vi "main.vi"() -> ()   [LabVIEW 2023] (continued)
     4245  0CF104A7   00000004    8        F0\t60\t22\tFC\tFF\tFF\tFF\t62\r\n      4244  0CF103A7   00000004    8        17\t1F\t08\t60\tB1\t1F\t08\t62\r\n      4244  0CF102A7   00000004    8        30\t75\tE0\t2E\t80\tFF\tFF\tFD\r\n      4243  0C3C4D4A   00000004    8        BE\tFF\tFF\t7F\t18\tFF\tFF\t62\r\n      4243  0CF101A7   00000004    8        68\t00\t97\tCC\t00\t19\t39\tEE\r\n      4242  18F120F0   00000004    8        2B\t75\t60\tB1\tB0\t01\tFF\tFF\r\n      4241  18F11FF0   00000004    8        FF\t3F\t90\t68\t88\t1B\t10\t2C\r\n      4232  1FFFFFFF   00000004    8        00\t20\tFF\tFF\tFF\tFF\tFF\tFF\r\n      4223  0CF102A7   00000004    8        30\t75\tE0\t2E\t80\tFF\tFF\tFD\r\n      4223  0CF101A7   00000004    8        68\t00\t97\tCC\t00\t19\t39\tED\r\n      4246  18F121F0   00000004    8        09\t34\t00\t00\tFF\tFF\tB0\t01\r\n      4245  18F106A7   00000004    8        00\tF7\tFF\tFF\tFF\tFF\tFF\tC5\r\n      4245  0CF104A7   00000004    8        F0\t60\t22\tFC\tFF\tFF\tFF\t62\r\n      4244  0CF103A7   00000004    8        17\t1F\t08\t60\tB1\t1F\t08\t62\r\n      4244  0CF102A7   00000004    8        30\t75\tE0\t2E\t80\tFF\tFF\tFD\r\n      4243  0C3C4D4A   00000004    8        BE\tFF\tFF\t7F\t18\tFF\tFF\t62\r\n      4243  0CF101A7   00000004    8        68\t00\t97\tCC\t00\t19\t39\tEE\r\n      4242  18F120F0   00000004    8        2B\t75\t60\tB1\tB0\t01\tFF\tFF\r\n      4241  18F11FF0   00000004    8        FF\t3F\t90\t68\t88\t1B\t10\t2C\r\n      4232  1FFFFFFF   00000004    8        00\t20\tFF\tFF\tFF\tFF\tFF\tFF\r\n      4223  0CF102A7   00000004    8        30\t75\tE0\t2E\t80\tFF\tFF\tFD\r\n      4247  1FFFFFFF   00000004    8        00\t00\tFF\tFF\tFF\tFF\tFF\tFF\r\n      4246  18F121F0   00000004    8        09\t34\t00\t00\tFF\tFF\tB0\t01\r\n      4245  18F106A7   00000004    8        00\tF7\tFF\tFF\tFF\tFF\tFF\tC5\r\n      4245  0CF104A7   00000004    8        F0\t60\t22\tFC\tFF\tFF\tFF\t62\r\n      4244  0CF103A7   00000004    8        17\t1F\t08\t60\tB1\t1F\t08\t62\r\n      4244  0CF102A7   00000004    8        30\t75\tE0\t2E\t80\tFF\tFF\tFD\r\n      4243  0C3C4D4A   00000004    8        BE\tFF\tFF\t7F\t18\tFF\tFF\t62\r\n      4243  0CF101A7   00000004    8        68\t00\t97\tCC\t00\t19\t39\tEE\r\n      4242  18F120F0   00000004    8        2B\t75\t60\tB1\tB0\t01\tFF\tFF\r\n      4241  18F11FF0   00000004    8        FF\t3F\t90\t68\t88\t1B\t10\t2C\r\n      4232  1FFFFFFF   00000004    8        00\t20\tFF\tFF\tFF\tFF\tFF\tFF\r\n      4252  1FFFFFFF   00000004    8        00\t20\tFF\tFF\tFF\tFF\tFF\tFF\r\n      4247  1FFFFFFF   00000004    8        00\t00\tFF\tFF\tFF\tFF\tFF\tFF\r\n      4246  18F121F0   00000004    8        09\t34\t00\t00\tFF\tFF\tB0\t01\r\n      4245  18F106A7   00000004    8        00\tF7\tFF\tFF\tFF\tFF\tFF\tC5\r\n      4245  0CF104A7   00000004    8        F0\t60\t22\tFC\tFF\tFF\tFF\t62\r\n      4244  0CF103A7   00000004    8        17\t1F\t08\t60\tB1\t1F\t08\t62\r\n      4244  0CF102A7   00000004    8        30\t75\tE0\t2E\t80\tFF\tFF\tFD\r\n      4243  0C3C4D4A   00000004    8        BE\tFF\tFF\t7F\t18\tFF\tFF\t62\r\n      4243  0CF101A7   00000004    8        68\t00\t97\tCC\t00\t19\t39\tEE\r\n      4242  18F120F0   00000004    8        2B\t75\t60\tB1\tB0\t01\tFF\tFF\r\n      4241  18F11FF0   00000004    8        FF\t3F\t90\t68\t88\t1B\t10\t2C\r\n      4262  1FFFFFFF   00000004    8        00\t20\tFF\tFF\tFF\tFF\tFF\tFF\r\n      4252  1FFFFFFF   00000004    8        00\t20\tFF\tFF\tFF\tFF\tFF\tFF\r\n      4247  1FFFFFFF   00000004    8        00\t00\tFF\tFF\tFF\tFF\tFF\tFF\r\n      4246  18F121F0   00000004    8        09\t34\t00\t00\tFF\tFF\tB0\t01\r\n      4245  18F106A7   00000004    8        00\tF7\tFF\tFF\tFF\tFF\tFF\tC5\r\n      4245  0CF104A7   00000004    8        F0\t60\t22\tFC\tFF\tFF\tFF\t62\r\n      4244  0CF103A7   00000004    8        17\t1F\t08\t60\tB1\t1F\t08\t62\r\n      4244  0CF102A7   00000004    8        30\t75\tE0\t2E\t80\tFF\tFF\tFD\r\n      4243  0C3C4D4A   00000004    8        BE\tFF\tFF\t7F\t18\tFF\tFF\t62\r\n      4243  0CF101A7   00000004    8        68\t00\t97\tCC\t00\t19\t39\tEE\r\n      4242  18F120F0   00000004    8        2B\t75\t60\tB1\tB0\t01\tFF\tFF\r\n      4263  0CF101A7   00000004    8        68\t00\t97\tCC\t00\t19\t39\tEF\r\n      4262  1FFFFFFF   00000004    8        00\t20\tFF\tFF\tFF\tFF\tFF\tFF\r\n      4252  1FFFFFFF   00000004    8        00\t20\tFF\tFF\tFF\tFF\tFF\tFF\r\n      4247  1FFFFFFF   00000004    8        00\t00\tFF\tFF\tFF\tFF\tFF\tFF\r\n      4246  18F121F0   00000004    8        09\t34\t00\t00\tFF\tFF\tB0\t01\r\n      4245  18F106A7   00000004    8        00\tF7\tFF\tFF\tFF\tFF\tFF\tC5\r\n      4245  0CF104A7   00000004    8        F0\t60\t22\tFC\tFF\tFF\tFF\t62\r\n      4244  0CF103A7   00000004    8        17\t1F\t08\t60\tB1\t1F\t08\t62\r\n      4244  0CF102A7   00000004    8        30\t75\tE0\t2E\t80\tFF\tFF\tFD\r\n      4243  0C3C4D4A   00000004    8        BE\tFF\tFF\t7F\t18\tFF\tFF\t62\r\n      4243  0CF101A7   00000004    8        68\t00\t97\tCC\t00\t19\t39\tEE\r\n      4263  0CF102A7   00000004    8        30\t75\tE0\t2E\t80\tFF\tFF\tFD\r\n      4263  0CF101A7   00000004    8        68\t00\t97\tCC\t00\t19\t39\tEF\r\n      4262  1FFFFFFF   00000004    8        00\t20\tFF\tFF\tFF\tFF\tFF\tFF\r\n      4252  1FFFFFFF   00000004    8        00\t20\tFF\tFF\tFF\tFF\tFF\tFF\r\n      4247  1FFFFFFF   00000004    8        00\t00\tFF\tFF\tFF\tFF\tFF\tFF\r\n      4246  18F121F0   00000004    8        09\t34\t00\t00\tFF\tFF\tB0\t01\r\n      4245  18F106A7   00000004    8        00\tF7\tFF\tFF\tFF\tFF\tFF\tC5\r\n      4245  0CF104A7   00000004    8        F0\t60\t22\tFC\tFF\tFF\tFF\t62\r\n      4244  0CF103A7   00000004    8        17\t1F\t08\t60\tB1\t1F\t08\t62\r\n      4244  0CF102A7   00000004    8        30\t75\tE0\t2E\t80\tFF\tFF\tFD\r\n      4243  0C3C4D4A   00000004    8        BE\tFF\tFF\t7F\t18\tFF\tFF\t62\r\n      4272  1FFFFFFF   00000004    8        00\t00\tFF\tFF\tFF\tFF\tFF\tFF\r\n      4263  0CF102A7   00000004    8        30\t75\tE0\t2E\t80\tFF\tFF\tFD\r\n      4263  0CF101A7   00000004    8        68\t00\t97\tCC\t00\t19\t39\tEF\r\n      4262  1FFFFFFF   00000004    8        00\t20\tFF\tFF\tFF\tFF\tFF\tFF\r\n      4252  1FFFFFFF   00000004    8        00\t20\tFF\tFF\tFF\tFF\tFF\tFF\r\n      4247  1FFFFFFF   00000004    8        00\t00\tFF\tFF\tFF\tFF\tFF\tFF\r\n      4246  18F121F0   00000004    8        09\t34\t00\t00\tFF\tFF\tB0\t01\r\n      4245  18F106A7   00000004    8        00\tF7\tFF\tFF\tFF\tFF\tFF\tC5\r\n      4245  0CF104A7   00000004    8        F0\t60\t22\tFC\tFF\tFF\tFF\t62\r\n      4244  0CF103A7   00000004    8        17\t1F\t08\t60\tB1\t1F\t08\t62\r\n      4244  0CF102A7   00000004    8        30\t75\tE0\t2E\t80\tFF\tFF\tFD\r\n      4282  1FFFFFFF   00000004    8        00\t00\tFF\tFF\tFF\tFF\tFF\tFF\r\n      4272  1FFFFFFF   00000004    8        00\t00\tFF\tFF\tFF\tFF\tFF\tFF\r\n      4263  0CF102A7   00000004    8        30\t75\tE0\t2E\t80\tFF\tFF\tFD\r\n      4263  0CF101A7   00000004    8        68\t00\t97\tCC\t00\t19\t39\tEF\r\n      4262  1FFFFFFF   00000004    8        00\t20\tFF\tFF\tFF\tFF\tFF\tFF\r\n      4252  1FFFFFFF   00000004    8        00\t20\tFF\tFF\tFF\tFF\tFF\tFF\r\n      4247  1FFFFFFF   00000004    8        00\t00\tFF\tFF\tFF\tFF\tFF\tFF\r\n      4246  18F121F0   00000004    8        09\t34\t00\t00\tFF\tFF\tB0\t01\r\n      4245  18F106A7   00000004    8        00\tF7\tFF\tFF\tFF\tFF\tFF\tC5\r\n      4245  0CF104A7   00000004    8        F0\t60\t22\tFC\tFF\tFF\tFF\t62\r\n      4244  0CF103A7   00000004    8        17\t1F\t08\t60\tB1\t1F\t08\t62\r\n      4283  0CF101A7   00000004    8        68\t00\t97\tCC\t00\t19\t39\tF0\r\n      4282  1FFFFFFF   00000004    8        00\t00\tFF\tFF\tFF\tFF\tFF\tFF\r\n      4272  1FFFFFFF   00000004    8        00\t00\tFF\tFF\tFF\tFF\tFF\tFF\r\n      4263  0CF102A7   00000004    8        30\t75\tE0\t2E\t80\tFF\tFF\tFD\r\n      4263  0CF101A7   00000004    8        68\t00\t97\tCC\t00\t19\t39\tEF\r\n      4262  1FFFFFFF   00000004    8        00\t20\tFF\tFF\tFF\tFF\tFF\tFF\r\n      4252  1FFFFFFF   00000004    8        00\t20\tFF\tFF\tFF\tFF\tFF\tFF\r\n      4247  1FFFFFFF   00000004    8        00\t00\tFF\tFF\tFF\tFF\tFF\tFF\r\n      4246  18F121F0   00000004    8        09\t34\t00\t00\tFF\tFF\tB0\t01\r\n      4245  18F106A7   00000004    8        00\tF7\tFF\tFF\tFF\tFF\tFF\tC5\r\n      4245  0CF104A7   00000004    8        F0\t60\t22\tFC\tFF\tFF\tFF\t62\r\n      4283  0CF102A7   00000004    8        30\t75\tE0\t2E\t80\tFF\tFF\tFD\r\n      4283  0CF101A7   00000004    8        68\t00\t97\tCC\t00\t19\t39\tF0\r\n      4282  1FFFFFFF   00000004    8        00\t00\tFF\tFF\tFF\tFF\tFF\tFF\r\n      4272  1FFFFFFF   00000004    8        00\t00\tFF\tFF\tFF\tFF\tFF\tFF\r\n      4263  0CF102A7   00000004    8        30\t75\tE0\t2E\t80\tFF\tFF\tFD\r\n      4263  0CF101A7   00000004    8        68\t00\t97\tCC\t00\t19\t39\tEF\r\n      4262  1FFFFFFF   00000004    8        00\t20\tFF\tFF\tFF\tFF\tFF\tFF\r\n      4252  1FFFFFFF   00000004    8        00\t20\tFF\tFF\tFF\tFF\tFF\tFF\r\n      4247  1FFFFFFF   00000004    8        00\t00\tFF\tFF\tFF\tFF\tFF\tFF\r\n      4246  18F121F0   00000004    8        09\t34\t00\t00\tFF\tFF\tB0\t01\r\n      4245  18F106A7   00000004    8        00\tF7\tFF\tFF\tFF\tFF\tFF\tC5\r\n      4292  1FFFFFFF   00000004    8        00\t20\tFF\tFF\tFF\tFF\tFF\tFF\r\n      4283  0CF102A7   00000004    8        30\t75\tE0\t2E\t80\tFF\tFF\tFD\r\n      4283  0CF101A7   00000004    8        68\t00\t97\tCC\t00\t19\t39\tF0\r\n      4282  1FFFFFFF   00000004    8        00\t00\tFF\tFF\tFF\tFF\tFF\tFF\r\n      4272  1FFFFFFF   00000004    8        00\t00\tFF\tFF\tFF\tFF\tFF\tFF\r\n      4263  0CF102A7   00000004    8        30\t75\tE0\t2E\t80\tFF\tFF\tFD\r\n      4263  0CF101A7   00000004    8        68\t00\t97\tCC\t00\t19\t39\tEF\r\n      4262  1FFFFFFF   00000004    8        00\t20\tFF\tFF\tFF\tFF\tFF\tFF\r\n      4252  1FFFFFFF   00000004    8        00\t20\tFF\tFF\tFF\tFF\tFF\tFF\r\n      4247  1FFFFFFF   00000004    8        00\t00\tFF\tFF\tFF\tFF\tFF\tFF\r\n      4246  18F121F0   00000004    8        09\t34\t00\t00\tFF\tFF\tB0\t01\r\n      4293  18F106A7   00000004    8        00\tF7\tFF\tFF\tFF\tFF\tFF\tC6\r\n      4292  1FFFFFFF   00000004    8        00\t20\tFF\tFF\tFF\tFF\tFF\tFF\r\n      4283  0CF102A7   00000004    8        30\t75\tE0\t2E\t80\tFF\tFF\tFD\r\n      4283  0CF101A7   00000004    8        68\t00\t97\tCC\t00\t19\t39\tF0\r\n      4282  1FFFFFFF   00000004    8        00\t00\tFF\tFF\tFF\tFF\tFF\tFF\r\n      4272  1FFFFFFF   00000004    8        00\t00\tFF\tFF\tFF\tFF\tFF\tFF\r\n      4263  0CF102A7   00000004    8        30\t75\tE0\t2E\t80\tFF\tFF\tFD\r\n      4263  0CF101A7   00000004    8        68\t00\t97\tCC\t00\t19\t39\tEF\r\n      4262  1FFFFFFF   00000004    8        00\t20\tFF\tFF\tFF\tFF\tFF\tFF\r\n      4252  1FFFFFFF   00000004    8        00\t20\tFF\tFF\tFF\tFF\tFF\tFF\r\n      4247  1FFFFFFF   00000004    8        00\t00\tFF\tFF\tFF\tFF\tFF\tFF\r\n      4302  1FFFFFFF   00000004    8        00\t00\tFF\tFF\tFF\tFF\tFF\tFF\r\n      4293  18F106A7   00000004    8        00\tF7\tFF\tFF\tFF\tFF\tFF\tC6\r\n      4292  1FFFFFFF   00000004    8        00\t20\tFF\tFF\tFF\tFF\tFF\tFF\r\n      4283  0CF102A7   00000004    8        30\t75\tE0\t2E\t80\tFF\tFF\tFD\r\n      4283  0CF101A7   00000004    8        68\t00\t97\tCC\t00\t19\t39\tF0\r\n      4282  1FFFFFFF   00000004    8        00\t00\tFF\tFF\tFF\tFF\tFF\tFF\r\n      4272  1FFFFFFF   00000004    8        00\t00\tFF\tFF\tFF\tFF\tFF\tFF\r\n      4263  0CF102A7   00000004    8        30\t75\tE0\t2E\t80\tFF\tFF\tFD\r\n      4263  0CF101A7   00000004    8        68\t00\t97\tCC\t00\t19\t39\tEF\r\n      4262  1FFFFFFF   00000004    8        00\t20\tFF\tFF\tFF\tFF\tFF\tFF\r\n      4252  1FFFFFFF   00000004    8        00\t20\tFF\tFF\tFF\tFF\tFF\tFF\r\n      4303  0CF101A7   00000004    8        68\t00\t97\tCC\t00\t19\t39\tF1\r\n      4302  1FFFFFFF   00000004    8        00\t00\tFF\tFF\tFF\tFF\tFF\tFF\r\n      4293  18F106A7   00000004    8        00\tF7\tFF\tFF\tFF\tFF\tFF\tC6\r\n      4292  1FFFFFFF   00000004    8        00\t20\tFF\tFF\tFF\tFF\tFF\tFF\r\n      4283  0CF102A7   00000004    8        30\t75\tE0\t2E\t80\tFF\tFF\tFD\r\n      4283  0CF101A7   00000004    8        68\t00\t97\tCC\t00\t19\t39\tF0\r\n      4282  1FFFFFFF   00000004    8        00\t00\tFF\tFF\tFF\tFF\tFF\tFF\r\n      4272  1FFFFFFF   00000004    8        00\t00\tFF\tFF\tFF\tFF\tFF\tFF\r\n      4263  0CF102A7   00000004    8        30\t75\tE0\t2E\t80\tFF\tFF\tFD\r\n      4263  0CF101A7   00000004    8        68\t00\t97\tCC\t00\t19\t39\tEF\r\n      4262  1FFFFFFF   00000004    8        00\t20\tFF\tFF\tFF\tFF\tFF\tFF\r\n      4303  0CF102A7   00000004    8        30\t75\tE0\t2E\t80\tFF\tFF\tFD\r\n      4303  0CF101A7   00000004    8        68\t00\t97\tCC\t00\t19\t39\tF1\r\n      4302  1FFFFFFF   00000004    8        00\t00\tFF\tFF\tFF\tFF\tFF\tFF\r\n      4293  18F106A7   00000004    8        00\tF7\tFF\tFF\tFF\tFF\tFF\tC6\r\n      4292  1FFFFFFF   00000004    8        00\t20\tFF\tFF\tFF\tFF\tFF\tFF\r\n      4283  0CF102A7   00000004    8        30\t75\tE0\t2E\t80\tFF\tFF\tFD\r\n      4283  0CF101A7   00000004    8        68\t00\t97\tCC\t00\t19\t39\tF0\r\n      4282  1FFFFFFF   00000004    8        00\t00\tFF\tFF\tFF\tFF\tFF\tFF\r\n      4272  1FFFFFFF   00000004    8        00\t00\tFF\tFF\tFF\tFF\tFF\tFF\r\n      4263  0CF102A7   00000004    8        30\t75\tE0\t2E\t80\tFF\tFF\tFD\r\n      4263  0CF101A7   00000004    8        68\t00\t97\tCC\t00\t19\t39\tEF\r\n      4312  1FFFFFFF   00000004    8        00\t20\tFF\tFF\tFF\tFF\tFF\tFF\r\n      4303  0CF102A7   00000004    8        30\t75\tE0\t2E\t80\tFF\tFF\tFD\r\n      4303  0CF101A7   00000004    8        68\t00\t97\tCC\t00\t19\t39\tF1\r\n      4302  1FFFFFFF   00000004    8        00\t00\tFF\tFF\tFF\tFF\tFF\tFF\r\n      4293  18F106A7   00000004    8        00\tF7\tFF\tFF\tFF\tFF\tFF\tC6\r\n      4292  1FFFFFFF   00000004    8        00\t20\tFF\tFF\tFF\tFF\tFF\tFF\r\n      4283  0CF102A7   00000004    8        30\t75\tE0\t2E\t80\tFF\tFF\tFD\r\n      4283  0CF101A7   00000004    8        68\t00\t97\tCC\t00\t19\t39\tF0\r\n      4282  1FFFFFFF   00000004    8        00\t00\tFF\tFF\tFF\tFF\tFF\tFF\r\n      4272  1FFFFFFF   00000004    8        00\t00\tFF\tFF\tFF\tFF\tFF\tFF\r\n      4263  0CF102A7   00000004    8        30\t75\tE0\t2E\t80\tFF\tFF\tFD\r\n      4322  1FFFFFFF   00000004    8        00\t00\tFF\tFF\tFF\tFF\tFF\tFF\r\n      4312  1FFFFFFF   00000004    8        00\t20\tFF\tFF\tFF\tFF\tFF\tFF\r\n      4303  0CF102A7   00000004    8        30\t75\tE0\t2E\t80\tFF\tFF\tFD\r\n      4303  0CF101A7   00000004    8        68\t00\t97\tCC\t00\t19\t39\tF1\r\n      4302  1FFFFFFF   00000004    8        00\t00\tFF\tFF\tFF\tFF\tFF\tFF\r\n      4293  18F106A7   00000004    8        00\tF7\tFF\tFF\tFF\tFF\tFF\tC6\r\n      4292  1FFFFFFF   00000004    8        00\t20\tFF\tFF\tFF\tFF\tFF\tFF\r\n      4283  0CF102A7   00000004    8        30\t75\tE0\t2E\t80\tFF\tFF\tFD\r\n      4283  0CF101A7   00000004    8        68\t00\t97\tCC\t00\t19\t39\tF0\r\n      4282  1FFFFFFF   00000004    8        00\t00\tFF\tFF\tFF\tFF\tFF\tFF\r\n      4272  1FFFFFFF   00000004    8        00\t00\tFF\tFF\tFF\tFF\tFF\tFF\r\n      4322  0CF101A7   00000004    8        68\t00\t97\tCC\t00\t19\t39\tF2\r\n      4322  1FFFFFFF   00000004    8        00\t00\tFF\tFF\tFF\tFF\tFF\tFF\r\n      4312  1FFFFFFF   00000004    8        00\t20\tFF\tFF\tFF\tFF\tFF\tFF\r\n      4303  0CF102A7   00000004    8        30\t75\tE0\t2E\t80\tFF\tFF\tFD\r\n      4303  0CF101A7   00000004    8        68\t00\t97\tCC\t00\t19\t39\tF1\r\n      4302  1FFFFFFF   00000004    8        00\t00\tFF\tFF\tFF\tFF\tFF\tFF\r\n      4293  18F106A7   00000004    8        00\tF7\tFF\tFF\tFF\tFF\tFF\tC6\r\n      4292  1FFFFFFF   00000004    8        00\t20\tFF\tFF\tFF\tFF\tFF\tFF\r\n      4283  0CF102A7   00000004    8        30\t75\tE0\t2E\t80\tFF\tFF\tFD\r\n      4283  0CF101A7   00000004    8        68\t00\t97\tCC\t00\t19\t39\tF0\r\n      4282  1FFFFFFF   00000004    8        00\t00\tFF\tFF\tFF\tFF\tFF\tFF\r\n      4323  0CF102A7   00000004    8        30\t75\tE0\t2E\t80\tFF\tFF\tFD\r\n      4322  0CF101A7   00000004    8        68\t00\t97\tCC\t00\t19\t39\tF2\r\n      4322  1FFFFFFF   00000004    8        00\t00\tFF\tFF\tFF\tFF\tFF\tFF\r\n      4312  1FFFFFFF   00000004    8        00\t20\tFF\tFF\tFF\tFF\tFF\tFF\r\n      4303  0CF102A7   00000004    8        30\t75\tE0\t2E\t80\tFF\tFF\tFD\r\n      4303  0CF101A7   00000004    8        68\t00\t97\tCC\t00\t19\t39\tF1\r\n      4302  1FFFFFFF   00000004    8        00\t00\tFF\tFF\tFF\tFF\tFF\tFF\r\n      4293  18F106A7   00000004    8        00\tF7\tFF\tFF\tFF\tFF\tFF\tC6\r\n      4292  1FFFFFFF   00000004    8        00\t20\tFF\tFF\tFF\tFF\tFF\tFF\r\n      4283  0CF102A7   00000004    8        30\t75\tE0\t2E\t80\tFF\tFF\tFD\r\n      4283  0CF101A7   00000004    8        68\t00\t97\tCC\t00\t19\t39\tF0\r\n      4332  1FFFFFFF   00000004    8        00\t20\tFF\tFF\tFF\tFF\tFF\tFF\r\n      4323  0CF102A7   00000004    8        30\t75\tE0\t2E\t80\tFF\tFF\tFD\r\n      4322  0CF101A7   00000004    8        68\t00\t97\tCC\t00\t19\t39\tF2\r\n      4322  1FFFFFFF   00000004    8        00\t00\tFF\tFF\tFF\tFF\tFF\tFF\r\n      4312  1FFFFFFF   00000004    8        00\t20\tFF\tFF\tFF\tFF\tFF\tFF\r\n      4303  0CF102A7   00000004    8        30\t75\tE0\t2E\t80\tFF\tFF\tFD\r\n      4303  0CF101A7   00000004    8        68\t00\t97\tCC\t00\t19\t39\tF1\r\n      4302  1FFFFFFF   00000004    8        00\t00\tFF\tFF\tFF\tFF\tFF\tFF\r\n      4293  18F106A7   00000004    8        00\tF7\tFF\tFF\tFF\tFF\tFF\tC6\r\n      4292  1FFFFFFF   00000004    8        00\t20\tFF\tFF\tFF\tFF\tFF\tFF\r\n      4283  0CF102A7   00000004    8        30\t75\tE0\t2E\t80\tFF\tFF\tFD\r\n      4341  18F11FF0   00000004    8        FF\t3F\t90\t68\t88\t1B\t10\t3C\r\n      4332  1FFFFFFF   00000004    8        00\t20\tFF\tFF\tFF\tFF\tFF\tFF\r\n      4323  0CF102A7   00000004    8        30\t75\tE0\t2E\t80\tFF\tFF\tFD\r\n      4322  0CF101A7   00000004    8        68\t00\t97\tCC\t00\t19\t39\tF2\r\n      4322  1FFFFFFF   00000004    8        00\t00\tFF\tFF\tFF\tFF\tFF\tFF\r\n      4312  1FFFFFFF   00000004    8        00\t20\tFF\tFF\tFF\tFF\tFF\tFF\r\n      4303  0CF102A7   00000004    8        30\t75\tE0\t2E\t80\tFF\tFF\tFD\r\n      4303  0CF101A7   00000004    8        68\t00\t97\tCC\t00\t19\t39\tF1\r\n      4302  1FFFFFFF   00000004    8        00\t00\tFF\tFF\tFF\tFF\tFF\tFF\r\n      4293  18F106A7   00000004    8        00\tF7\tFF\tFF\tFF\tFF\tFF\tC6\r\n      4292  1FFFFFFF   00000004    8        00\t20\tFF\tFF\tFF\tFF\tFF\tFF\r\n      4342  18F120F0   00000004    8        2B\t75\t60\tB1\tB0\t01\tFF\tFF\r\n      4341  18F11FF0   00000004    8        FF\t3F\t90\t68\t88\t1B\t10\t3C\r\n      4332  1FFFFFFF   00000004    8        00\t20\tFF\tFF\tFF\tFF\tFF\tFF\r\n      4323  0CF102A7   00000004    8        30\t75\tE0\t2E\t80\tFF\tFF\tFD\r\n      4322  0CF101A7   00000004    8        68\t00\t97\tCC\t00\t19\t39\tF2\r\n      4322  1FFFFFFF   00000004    8        00\t00\tFF\tFF\tFF\tFF\tFF\tFF\r\n      4312  1FFFFFFF   00000004    8        00\t20\tFF\tFF\tFF\tFF\tFF\tFF\r\n      4303  0CF102A7   00000004    8        30\t75\tE0\t2E\t80\tFF\tFF\tFD\r\n      4303  0CF101A7   00000004    8        68\t00\t97\tCC\t00\t19\t39\tF1\r\n      4302  1FFFFFFF   00000004    8        00\t00\tFF\tFF\tFF\tFF\tFF\tFF\r\n      4293  18F106A7   00000004    8        00\tF7\tFF\tFF\tFF\tFF\tFF\tC6\r\n      4343  0CF101A7   00000004    8        68\t00\t97\tCC\t00\t19\t39\tF3\r\n      4342  18F120F0   00000004    8        2B\t75\t60\tB1\tB0\t01\tFF\tFF\r\n      4341  18F11FF0   00000004    8        FF\t3F\t90\t68\t88\t1B\t10\t3C\r\n      4332  1FFFFFFF   00000004    8        00\t20\tFF\tFF\tFF\tFF\tFF\tFF\r\n      4323  0CF102A7   00000004    8        30\t75\tE0\t2E\t80\tFF\tFF\tFD\r\n      4322  0CF101A7   00000004    8        68\t00\t97\tCC\t00\t19\t39\tF2\r\n      4322  1FFFFFFF   00000004    8        00\t00\tFF\tFF\tFF\tFF\tFF\tFF\r\n      4312  1FFFFFFF   00000004    8        00\t20\tFF\tFF\tFF\tFF\tFF\tFF\r\n      4303  0CF102A7   00000004    8        30\t75\tE0\t2E\t80\tFF\tFF\tFD\r\n      4303  0CF101A7   00000004    8        68\t00\t97\tCC\t00\t19\t39\tF1\r\n      4302  1FFFFFFF   00000004    8        00\t00\tFF\tFF\tFF\tFF\tFF\tFF\r\n      4343  0C3C4D4A   00000004    8        BE\tFF\tFF\t7F\t18\tFF\tFF\t63\r\n      4343  0CF101A7   00000004    8        68\t00\t97\tCC\t00\t19\t39\tF3\r\n      4342  18F120F0   00000004    8        2B\t75\t60\tB1\tB0\t01\tFF\tFF\r\n      4341  18F11FF0   00000004    8        FF\t3F\t90\t68\t88\t1B\t10\t3C\r\n      4332  1FFFFFFF   00000004    8        00\t20\tFF\tFF\tFF\tFF\tFF\tFF\r\n      4323  0CF102A7   00000004    8        30\t75\tE0\t2E\t80\tFF\tFF\tFD\r\n      4322  0CF101A7   00000004    8        68\t00\t97\tCC\t00\t19\t39\tF2\r\n      4322  1FFFFFFF   00000004    8        00\t00\tFF\tFF\tFF\tFF\tFF\tFF\r\n      4312  1FFFFFFF   00000004    8        00\t20\tFF\tFF\tFF\tFF\tFF\tFF\r\n      4303  0CF102A7   00000004    8        30\t75\tE0\t2E\t80\tFF\tFF\tFD\r\n      4303  0CF101A7   00000004    8        68\t00\t97\tCC\t00\t19\t39\tF1\r\n      4344  0CF102A7   00000004    8        30\t75\tE0\t2E\t80\tFF\tFF\tFD\r\n      4343  0C3C4D4A   00000004    8        BE\tFF\tFF\t7F\t18\tFF\tFF\t63\r\n      4343  0CF101A7   00000004    8        68\t00\t97\tCC\t00\t19\t39\tF3\r\n      4342  18F120F0   00000004    8        2B\t75\t60\tB1\tB0\t01\tFF\tFF\r\n      4341  18F11FF0   00000004    8        FF\t3F\t90\t68\t88\t1B\t10\t3C\r\n      4332  1FFFFFFF   00000004    8        00\t20\tFF\tFF\tFF\tFF\tFF\tFF\r\n      4323  0CF102A7   00000004    8        30\t75\tE0\t2E\t80\tFF\tFF\tFD\r\n      4322  0CF101A7   00000004    8        68\t00\t97\tCC\t00\t19\t39\tF2\r\n      4322  1FFFFFFF   00000004    8        00\t00\tFF\tFF\tFF\tFF\tFF\tFF\r\n      4312  1FFFFFFF   00000004    8        00\t20\tFF\tFF\tFF\tFF\tFF\tFF\r\n      4303  0CF102A7   00000004    8        30\t75\tE0\t2E\t80\tFF\tFF\tFD\r\n      4344  0CF103A7   00000004    8        17\t1F\t08\t60\tB1\t1F\t08\t63\r\n      4344  0CF102A7   00000004    8        30\t75\tE0\t2E\t80\tFF\tFF\tFD\r\n      4343  0C3C4D4A   00000004    8        BE\tFF\tFF\t7F\t18\tFF\tFF\t63\r\n      4343  0CF101A7   00000004    8        68\t00\t97\tCC\t00\t19\t39\tF3\r\n      4342  18F120F0   00000004    8        2B\t75\t60\tB1\tB0\t01\tFF\tFF\r\n      4341  18F11FF0   00000004    8        FF\t3F\t90\t68\t88\t1B\t10\t3C\r\n      4332  1FFFFFFF   00000004    8        00\t20\tFF\tFF\tFF\tFF\tFF\tFF\r\n      4323  0CF102A7   00000004    8        30\t75\tE0\t2E\t80\tFF\tFF\tFD\r\n      4322  0CF101A7   00000004    8        68\t00\t97\tCC\t00\t19\t39\tF2\r\n      4322  1FFFFFFF   00000004    8        00\t00\tFF\tFF\tFF\tFF\tFF\tFF\r\n      4312  1FFFFFFF   00000004    8        00\t20\tFF\tFF\tFF\tFF\tFF\tFF\r\n      4345  0CF104A7   00000004    8        F0\t60\t22\tFC\tFF\tFF\tFF\t63\r\n      4344  0CF103A7   00000004    8        17\t1F\t08\t60\tB1\t1F\t08\t63\r\n      4344  0CF102A7   00000004    8        30\t75\tE0\t2E\t80\tFF\tFF\tFD\r\n      4343  0C3C4D4A   00000004    8        BE\tFF\tFF\t7F\t18\tFF\tFF\t63\r\n      4343  0CF101A7   00000004    8        68\t00\t97\tCC\t00\t19\t39\tF3\r\n      4342  18F120F0   00000004    8        2B\t75\t60\tB1\tB0\t01\tFF\tFF\r\n      4341  18F11FF0   00000004    8        FF\t3F\t90\t68\t88\t1B\t10\t3C\r\n      4332  1FFFFFFF   00000004    8        00\t20\tFF\tFF\tFF\tFF\tFF\tFF\r\n      4323  0CF102A7   00000004    8        30\t75\tE0\t2E\t80\tFF\tFF\tFD\r\n      4322  0CF101A7   00000004    8        68\t00\t97\tCC\t00\t19\t39\tF2\r\n      4322  1FFFFFFF   00000004    8        00\t00\tFF\tFF\tFF\tFF\tFF\tFF\r\n      4345  18F106A7   00000004    8        00\tF7\tFF\tFF\tFF\tFF\tFF\tC7\r\n      4345  0CF104A7   00000004    8        F0\t60\t22\tFC\tFF\tFF\tFF\t63\r\n      4344  0CF103A7   00000004    8        17\t1F\t08\t60\tB1\t1F\t08\t63\r\n      4344  0CF102A7   00000004    8        30\t75\tE0\t2E\t80\tFF\tFF\tFD\r\n      4343  0C3C4D4A   00000004    8        BE\tFF\tFF\t7F\t18\tFF\tFF\t63\r\n      4343  0CF101A7   00000004    8        68\t00\t97\tCC\t00\t19\t39\tF3\r\n      4342  18F120F0   00000004    8        2B\t75\t60\tB1\tB0\t01\tFF\tFF\r\n      4341  18F11FF0   00000004    8        FF\t3F\t90\t68\t88\t1B\t10\t3C\r\n      4332  1FFFFFFF   00000004    8        00\t20\tFF\tFF\tFF\tFF\tFF\tFF\r\n      4323  0CF102A7   00000004    8        30\t75\tE0\t2E\t80\tFF\tFF\tFD\r\n      4322  0CF101A7   00000004    8        68\t00\t97\tCC\t00\t19\t39\tF2\r\n      4346  18F121F0   00000004    8        09\t34\t00\t00\tFF\tFF\tB0\t01\r\n      4345  18F106A7   00000004    8        00\tF7\tFF\tFF\tFF\tFF\tFF\tC7\r\n      4345  0CF104A7   00000004    8        F0\t60\t22\tFC\tFF\tFF\tFF\t63\r\n      4344  0CF103A7   00000004    8        17\t1F\t08\t60\tB1\t1F\t08\t63\r\n      4344  0CF102A7   00000004    8        30\t75\tE0\t2E\t80\tFF\tFF\tFD\r\n      4343  0C3C4D4A   00000004    8        BE\tFF\tFF\t7F\t18\tFF\tFF\t63\r\n      4343  0CF101A7   00000004    8        68\t00\t97\tCC\t00\t19\t39\tF3\r\n      4342  18F120F0   00000004    8        2B\t75\t60\tB1\tB0\t01\tFF\tFF\r\n      4341  18F11FF0   00000004    8        FF\t3F\t90\t68\t88\t1B\t10\t3C\r\n      4332  1FFFFFFF   00000004    8        00\t20\tFF\tFF\tFF\tFF\tFF\tFF\r\n      4323  0CF102A7   00000004    8        30\t75\tE0\t2E\t80\tFF\tFF\tFD\r\n      4346  1FFFFFFF   00000004    8        00\t20\tFF\tFF\tFF\tFF\tFF\tFF\r\n      4346  18F121F0   00000004    8        09\t34\t00\t00\tFF\tFF\tB0\t01\r\n      4345  18F106A7   00000004    8        00\tF7\tFF\tFF\tFF\tFF\tFF\tC7\r\n      4345  0CF104A7   00000004    8        F0\t60\t22\tFC\tFF\tFF\tFF\t63\r\n      4344  0CF103A7   00000004    8        17\t1F\t08\t60\tB1\t1F\t08\t63\r\n      4344  0CF102A7   00000004    8        30\t75\tE0\t2E\t80\tFF\tFF\tFD\r\n      4343  0C3C4D4A   00000004    8        BE\tFF\tFF\t7F\t18\tFF\tFF\t63\r\n      4343  0CF101A7   00000004    8        68\t00\t97\tCC\t00\t19\t39\tF3\r\n      4342  18F120F0   00000004    8        2B\t75\t60\tB1\tB0\t01\tFF\tFF\r\n      4341  18F11FF0   00000004    8        FF\t3F\t90\t68\t88\t1B\t10\t3C\r\n      4332  1FFFFFFF   00000004    8        00\t20\tFF\tFF\tFF\tFF\tFF\tFF\r\n      4352  1FFFFFFF   00000004    8        00\t00\tFF\tFF\tFF\tFF\tFF\tFF\r\n      4346  1FFFFFFF   00000004    8        00\t20\tFF\tFF\tFF\tFF\tFF\tFF\r\n      4346  18F121F0   00000004    8        09\t34\t00\t00\tFF\tFF\tB0\t01\r\n      4345  18F106A7   00000004    8        00\tF7\tFF\tFF\tFF\tFF\tFF\tC7\r\n      4345  0CF104A7   00000004    8        F0\t60\t22\tFC\tFF\tFF\tFF\t63\r\n      4344  0CF103A7   00000004    8        17\t1F\t08\t60\tB1\t1F\t08\t63\r\n      4344  0CF102A7   00000004    8        30\t75\tE0\t2E\t80\tFF\tFF\tFD\r\n      4343  0C3C4D4A   00000004    8        BE\tFF\tFF\t7F\t18\tFF\tFF\t63\r\n      4343  0CF101A7   00000004    8        68\t00\t97\tCC\t00\t19\t39\tF3\r\n      4342  18F120F0   00000004    8        2B\t75\t60\tB1\tB0\t01\tFF\tFF\r\n      4341  18F11FF0   00000004    8        FF\t3F\t90\t68\t88\t1B\t10\t3C\r\n      4362  1FFFFFFF   00000004    8        00\t00\tFF\tFF\tFF\tFF\tFF\tFF\r\n      4352  1FFFFFFF   00000004    8        00\t00\tFF\tFF\tFF\tFF\tFF\tFF\r\n      4346  1FFFFFFF   00000004    8        00\t20\tFF\tFF\tFF\tFF\tFF\tFF\r\n      4346  18F121F0   00000004    8        09\t34\t00\t00\tFF\tFF\tB0\t01\r\n      4345  18F106A7   00000004    8        00\tF7\tFF\tFF\tFF\tFF\tFF\tC7\r\n      4345  0CF104A7   00000004    8        F0\t60\t22\tFC\tFF\tFF\tFF\t63\r\n      4344  0CF103A7   00000004    8        17\t1F\t08\t60\tB1\t1F\t08\t63\r\n      4344  0CF102A7   00000004    8        30\t75\tE0\t2E\t80\tFF\tFF\tFD\r\n      4343  0C3C4D4A   00000004    8        BE\tFF\tFF\t7F\t18\tFF\tFF\t63\r\n      4343  0CF101A7   00000004    8        68\t00\t97\tCC\t00\t19\t39\tF3\r\n      4342  18F120F0   00000004    8        2B\t75\t60\tB1\tB0\t01\tFF\tFF\r\n      4363  0CF101A7   00000004    8        68\t00\t97\tCC\t00\t19\t39\tF4\r\n      4362  1FFFFFFF   00000004    8        00\t00\tFF\tFF\tFF\tFF\tFF\tFF\r\n      4352  1FFFFFFF   00000004    8        00\t00\tFF\tFF\tFF\tFF\tFF\tFF\r\n      4346  1FFFFFFF   00000004    8        00\t20\tFF\tFF\tFF\tFF\tFF\tFF\r\n      4346  18F121F0   00000004    8        09\t34\t00\t00\tFF\tFF\tB0\t01\r\n      4345  18F106A7   00000004    8        00\tF7\tFF\tFF\tFF\tFF\tFF\tC7\r\n      4345  0CF104A7   00000004    8        F0\t60\t22\tFC\tFF\tFF\tFF\t63\r\n      4344  0CF103A7   00000004    8        17\t1F\t08\t60\tB1\t1F\t08\t63\r\n      4344  0CF102A7   00000004    8        30\t75\tE0\t2E\t80\tFF\tFF\tFD\r\n      4343  0C3C4D4A   00000004    8        BE\tFF\tFF\t7F\t18\tFF\tFF\t63\r\n      4343  0CF101A7   00000004    8        68\t00\t97\tCC\t00\t19\t39\tF3\r\n      4363  0CF102A7   00000004    8        30\t75\tE0\t2E\t80\tFF\tFF\tFD\r\n      4363  0CF101A7   00000004    8        68\t00\t97\tCC\t00\t19\t39\tF4\r\n      4362  1FFFFFFF   00000004    8        00\t00\tFF\tFF\tFF\tFF\tFF\tFF\r\n      4352  1FFFFFFF   00000004    8        00\t00\tFF\tFF\tFF\tFF\tFF\tFF\r\n      4346  1FFFFFFF   00000004    8        00\t20\tFF\tFF\tFF\tFF\tFF\tFF\r\n      4346  18F121F0   00000004    8        09\t34\t00\t00\tFF\tFF\tB0\t01\r\n      4345  18F106A7   00000004    8        00\tF7\tFF\tFF\tFF\tFF\tFF\tC7\r\n      4345  0CF104A7   00000004    8        F0\t60\t22\tFC\tFF\tFF\tFF\t63\r\n      4344  0CF103A7   00000004    8        17\t1F\t08\t60\tB1\t1F\t08\t63\r\n      4344  0CF102A7   00000004    8        30\t75\tE0\t2E\t80\tFF\tFF\tFD\r\n      4343  0C3C4D4A   00000004    8        BE\tFF\tFF\t7F\t18\tFF\tFF\t63\r\n      4372  1FFFFFFF   00000004    8        00\t00\tFF\tFF\tFF\tFF\tFF\tFF\r\n      4363  0CF102A7   00000004    8        30\t75\tE0\t2E\t80\tFF\tFF\tFD\r\n      4363  0CF101A7   00000004    8        68\t00\t97\tCC\t00\t19\t39\tF4\r\n      4362  1FFFFFFF   00000004    8        00\t00\tFF\tFF\tFF\tFF\tFF\tFF\r\n      4352  1FFFFFFF   00000004    8        00\t00\tFF\tFF\tFF\tFF\tFF\tFF\r\n      4346  1FFFFFFF   00000004    8        00\t20\tFF\tFF\tFF\tFF\tFF\tFF\r\n      4346  18F121F0   00000004    8        09\t34\t00\t00\tFF\tFF\tB0\t01\r\n      4345  18F106A7   00000004    8        00\tF7\tFF\tFF\tFF\tFF\tFF\tC7\r\n      4345  0CF104A7   00000004    8        F0\t60\t22\tFC\tFF\tFF\tFF\t63\r\n      4344  0CF103A7   00000004    8        17\t1F\t08\t60\tB1\t1F\t08\t63\r\n      4344  0CF102A7   00000004    8        30\t75\tE0\t2E\t80\tFF\tFF\tFD\r\n      4382  1FFFFFFF   00000004    8        00\t00\tFF\tFF\tFF\tFF\tFF\tFF\r\n      4372  1FFFFFFF   00000004    8        00\t00\tFF\tFF\tFF\tFF\tFF\tFF\r\n      4363  0CF102A7   00000004    8        30\t75\tE0\t2E\t80\tFF\tFF\tFD\r\n      4363  0CF101A7   00000004    8        68\t00\t97\tCC\t00\t19\t39\tF4\r\n      4362  1FFFFFFF   00000004    8        00\t00\tFF\tFF\tFF\tFF\tFF\tFF\r\n      4352  1FFFFFFF   00000004    8        00\t00\tFF\tFF\tFF\tFF\tFF\tFF\r\n      4346  1FFFFFFF   00000004    8        00\t20\tFF\tFF\tFF\tFF\tFF\tFF\r\n      4346  18F121F0   00000004    8        09\t34\t00\t00\tFF\tFF\tB0\t01\r\n      4345  18F106A7   00000004    8        00\tF7\tFF\tFF\tFF\tFF\tFF\tC7\r\n      4345  0CF104A7   00000004    8        F0\t60\t22\tFC\tFF\tFF\tFF\t63\r\n      4344  0CF103A7   00000004    8        17\t1F\t08\t60\tB1\t1F\t08\t63\r\n      4382  0CF101A7   00000004    8        68\t00\t97\tCC\t00\t19\t39\tF5\r\n      4382  1FFFFFFF   00000004    8        00\t00\tFF\tFF\tFF\tFF\tFF\tFF\r\n      4372  1FFFFFFF   00000004    8        00\t00\tFF\tFF\tFF\tFF\tFF\tFF\r\n      4363  0CF102A7   00000004    8        30\t75\tE0\t2E\t80\tFF\tFF\tFD\r\n      4363  0CF101A7   00000004    8        68\t00\t97\tCC\t00\t19\t39\tF4\r\n      4362  1FFFFFFF   00000004    8        00\t00\tFF\tFF\tFF\tFF\tFF\tFF\r\n      4352  1FFFFFFF   00000004    8        00\t00\tFF\tFF\tFF\tFF\tFF\tFF\r\n      4346  1FFFFFFF   00000004    8        00\t20\tFF\tFF\tFF\tFF\tFF\tFF\r\n      4346  18F121F0   00000004    8        09\t34\t00\t00\tFF\tFF\tB0\t01\r\n      4345  18F106A7   00000004    8        00\tF7\tFF\tFF\tFF\tFF\tFF\tC7\r\n      4345  0CF104A7   00000004    8        F0\t60\t22\tFC\tFF\tFF\tFF\t63\r\n      4383  0CF102A7   00000004    8        30\t75\tE0\t2E\t80\tFF\tFF\tFD\r\n      4382  0CF101A7   00000004    8        68\t00\t97\tCC\t00\t19\t39\tF5\r\n      4382  1FFFFFFF   00000004    8        00\t00\tFF\tFF\tFF\tFF\tFF\tFF\r\n      4372  1FFFFFFF   00000004    8        00\t00\tFF\tFF\tFF\tFF\tFF\tFF\r\n      4363  0CF102A7   00000004    8        30\t75\tE0\t2E\t80\tFF\tFF\tFD\r\n      4363  0CF101A7   00000004    8        68\t00\t97\tCC\t00\t19\t39\tF4\r\n      4362  1FFFFFFF   00000004    8        00\t00\tFF\tFF\tFF\tFF\tFF\tFF\r\n      4352  1FFFFFFF   00000004    8        00\t00\tFF\tFF\tFF\tFF\tFF\tFF\r\n      4346  1FFFFFFF   00000004    8        00\t20\tFF\tFF\tFF\tFF\tFF\tFF\r\n      4346  18F121F0   00000004    8        09\t34\t00\t00\tFF\tFF\tB0\t01\r\n      4345  18F106A7   00000004    8        00\tF7\tFF\tFF\tFF\tFF\tFF\tC7\r\n      4392  1FFFFFFF   00000004    8        00\t00\tFF\tFF\tFF\tFF\tFF\tFF\r\n      4383  0CF102A7   00000004    8        30\t75\tE0\t2E\t80\tFF\tFF\tFD\r\n      4382  0CF101A7   00000004    8        68\t00\t97\tCC\t00\t19\t39\tF5\r\n      4382  1FFFFFFF   00000004    8        00\t00\tFF\tFF\tFF\tFF\tFF\tFF\r\n      4372  1FFFFFFF   00000004    8        00\t00\tFF\tFF\tFF\tFF\tFF\tFF\r\n      4363  0CF102A7   00000004    8        30\t75\tE0\t2E\t80\tFF\tFF\tFD\r\n      4363  0CF101A7   00000004    8        68\t00\t97\tCC\t00\t19\t39\tF4\r\n      4362  1FFFFFFF   00000004    8        00\t00\tFF\tFF\tFF\tFF\tFF\tFF\r\n      4352  1FFFFFFF   00000004    8        00\t00\tFF\tFF\tFF\tFF\tFF\tFF\r\n      4346  1FFFFFFF   00000004    8        00\t20\tFF\tFF\tFF\tFF\tFF\tFF\r\n      4346  18F121F0   00000004    8        09\t34\t00\t00\tFF\tFF\tB0\t01\r\n      4393  18F106A7   00000004    8        00\tF7\tFF\tFF\tFF\tFF\tFF\tC8\r\n      4392  1FFFFFFF   00000004    8        00\t00\tFF\tFF\tFF\tFF\tFF\tFF\r\n      4383  0CF102A7   00000004    8        30\t75\tE0\t2E\t80\tFF\tFF\tFD\r\n      4382  0CF101A7   00000004    8        68\t00\t97\tCC\t00\t19\t39\tF5\r\n      4382  1FFFFFFF   00000004    8        00\t00\tFF\tFF\tFF\tFF\tFF\tFF\r\n      4372  1FFFFFFF   00000004    8        00\t00\tFF\tFF\tFF\tFF\tFF\tFF\r\n      4363  0CF102A7   00000004    8        30\t75\tE0\t2E\t80\tFF\tFF\tFD\r\n      4363  0CF101A7   00000004    8        68\t00\t97\tCC\t00\t19\t39\tF4\r\n      4362  1FFFFFFF   00000004    8        00\t00\tFF\tFF\tFF\tFF\tFF\tFF\r\n      4352  1FFFFFFF   00000004    8        00\t00\tFF\tFF\tFF\tFF\tFF\tFF\r\n      4346  1FFFFFFF   00000004    8        00\t20\tFF\tFF\tFF\tFF\tFF\tFF\r\n      4402  1FFFFFFF   00000004    8        00\t00\tFF\tFF\tFF\tFF\tFF\tFF\r\n      4393  18F106A7   00000004    8        00\tF7\tFF\tFF\tFF\tFF\tFF\tC8\r\n      4392  1FFFFFFF   00000004    8        00\t00\tFF\tFF\tFF\tFF\tFF\tFF\r\n      4383  0CF102A7   00000004    8        30\t75\tE0\t2E\t80\tFF\tFF\tFD\r\n      4382  0CF101A7   00000004    8        68\t00\t97\tCC\t00\t19\t39\tF5\r\n      4382  1FFFFFFF   00000004    8        00\t00\tFF\tFF\tFF\tFF\tFF\tFF\r\n      4372  1FFFFFFF   00000004    8        00\t00\tFF\tFF\tFF\tFF\tFF\tFF\r\n      4363  0CF102A7   00000004    8        30\t75\tE0\t2E\t80\tFF\tFF\tFD\r\n      4363  0CF101A7   00000004    8        68\t00\t97\tCC\t00\t19\t39\tF4\r\n      4362  1FFFFFFF   00000004    8        00\t00\tFF\tFF\tFF\tFF\tFF\tFF\r\n      4352  1FFFFFFF   00000004    8        00\t00\tFF\tFF\tFF\tFF\tFF\tFF\r\n      4403  0CF101A7   00000004    8        68\t00\t97\tCC\t00\t19\t39\tF6\r\n      4402  1FFFFFFF   00000004    8        00\t00\tFF\tFF\tFF\tFF\tFF\tFF\r\n      4393  18F106A7   00000004    8        00\tF7\tFF\tFF\tFF\tFF\tFF\tC8\r\n      4392  1FFFFFFF   00000004    8        00\t00\tFF\tFF\tFF\tFF\tFF\tFF\r\n      4383  0CF102A7   00000004    8        30\t75\tE0\t2E\t80\tFF\tFF\tFD\r\n      4382  0CF101A7   00000004    8        68\t00\t97\tCC\t00\t19\t39\tF5\r\n      4382  1FFFFFFF   00000004    8        00\t00\tFF\tFF\tFF\tFF\tFF\tFF\r\n      4372  1FFFFFFF   00000004    8        00\t00\tFF\tFF\tFF\tFF\tFF\tFF\r\n      4363  0CF102A7   00000004    8        30\t75\tE0\t2E\t80\tFF\tFF\tFD\r\n      4363  0CF101A7   00000004    8        68\t00\t97\tCC\t00\t19\t39\tF4\r\n      4362  1FFFFFFF   00000004    8        00\t00\tFF\tFF\tFF\tFF\tFF\tFF\r\n      4403  0CF102A7   00000004    8        30\t75\tE0\t2E\t80\tFF\tFF\tFD\r\n      4403  0CF101A7   00000004    8        68\t00\t97\tCC\t00\t19\t39\tF6\r\n      4402  1FFFFFFF   00000004    8        00\t00\tFF\tFF\tFF\tFF\tFF\tFF\r\n      4393  18F106A7   00000004    8        00\tF7\tFF\tFF\tFF\tFF\tFF\tC8\r\n      4392  1FFFFFFF   00000004    8        00\t00\tFF\tFF\tFF\tFF\tFF\tFF\r\n      4383  0CF102A7   00000004    8        30\t75\tE0\t2E\t80\tFF\tFF\tFD\r\n      4382  0CF101A7   00000004    8        68\t00\t97\tCC\t00\t19\t39\tF5\r\n      4382  1FFFFFFF   00000004    8        00\t00\tFF\tFF\tFF\tFF\tFF\tFF\r\n      4372  1FFFFFFF   00000004    8        00\t00\tFF\tFF\tFF\tFF\tFF\tFF\r\n      4363  0CF102A7   00000004    8        30\t75\tE0\t2E\t80\tFF\tFF\tFD\r\n      4363  0CF101A7   00000004    8        68\t00\t97\tCC\t00\t19\t39\tF4\r\n      4412  1FFFFFFF   00000004    8        00\t00\tFF\tFF\tFF\tFF\tFF\tFF\r\n      4403  0CF102A7   00000004    8        30\t75\tE0\t2E\t80\tFF\tFF\tFD\r\n      4403  0CF101A7   00000004    8        68\t00\t97\tCC\t00\t19\t39\tF6\r\n      4402  1FFFFFFF   00000004    8        00\t00\tFF\tFF\tFF\tFF\tFF\tFF\r\n      4393  18F106A7   00000004    8        00\tF7\tFF\tFF\tFF\tFF\tFF\tC8\r\n      4392  1FFFFFFF   00000004    8        00\t00\tFF\tFF\tFF\tFF\tFF\tFF\r\n      4383  0CF102A7   00000004    8        30\t75\tE0\t2E\t80\tFF\tFF\tFD\r\n      4382  0CF101A7   00000004    8        68\t00\t97\tCC\t00\t19\t39\tF5\r\n      4382  1FFFFFFF   00000004    8        00\t00\tFF\tFF\tFF\tFF\tFF\tFF\r\n      4372  1FFFFFFF   00000004    8        00\t00\tFF\tFF\tFF\tFF\tFF\tFF\r\n      4363  0CF102A7   00000004    8        30\t75\tE0\t2E\t80\tFF\tFF\tFD\r\n      4422  1FFFFFFF   00000004    8        00\t00\tFF\tFF\tFF\tFF\tFF\tFF\r\n      4412  1FFFFFFF   00000004    8        00\t00\tFF\tFF\tFF\tFF\tFF\tFF\r\n      4403  0CF102A7   00000004    8        30\t75\tE0\t2E\t80\tFF\tFF\tFD\r\n      4403  0CF101A7   00000004    8        68\t00\t97\tCC\t00\t19\t39\tF6\r\n      4402  1FFFFFFF   00000004    8        00\t00\tFF\tFF\tFF\tFF\tFF\tFF\r\n      4393  18F106A7   00000004    8        00\tF7\tFF\tFF\tFF\tFF\tFF\tC8\r\n      4392  1FFFFFFF   00000004    8        00\t00\tFF\tFF\tFF\tFF\tFF\tFF\r\n      4383  0CF102A7   00000004    8        30\t75\tE0\t2E\t80\tFF\tFF\tFD\r\n      4382  0CF101A7   00000004    8        68\t00\t97\tCC\t00\t19\t39\tF5\r\n      4382  1FFFFFFF   00000004    8        00\t00\tFF\tFF\tFF\tFF\tFF\tFF\r\n      4372  1FFFFFFF   00000004    8        00\t00\tFF\tFF\tFF\tFF\tFF\tFF\r\n      4423  0CF101A7   00000004    8        68\t00\t97\tCC\t00\t19\t39\tF7\r\n      4422  1FFFFFFF   00000004    8        00\t00\tFF\tFF\tFF\tFF\tFF\tFF\r\n      4412  1FFFFFFF   00000004    8        00\t00\tFF\tFF\tFF\tFF\tFF\tFF\r\n      4403  0CF102A7   00000004    8        30\t75\tE0\t2E\t80\tFF\tFF\tFD\r\n      4403  0CF101A7   00000004    8        68\t00\t97\tCC\t00\t19\t39\tF6\r\n      4402  1FFFFFFF   00000004    8        00\t00\tFF\tFF\tFF\tFF\tFF\tFF\r\n      4393  18F106A7   00000004    8        00\tF7\tFF\tFF\tFF\tFF\tFF\tC8\r\n      4392  1FFFFFFF   00000004    8        00\t00\tFF\tFF\tFF\tFF\t
